vi "nejistota_A.vi"(11 "Array":dbl[](array[numeric])) -> (2 "nejistota_A":dbl, 3 "mean":dbl)   [LabVIEW 2022 SP3]
uses:
  <vilib>/Analysis/baseanly.llb/Mean (DBL).vi
  <vilib>/Analysis/NI_AALBase.lvlib
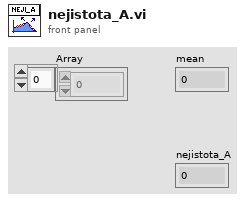
[diagram p1: front panel]
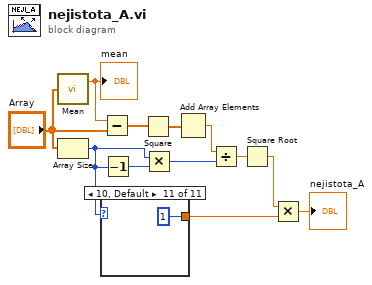
[diagram p0: block diagram]
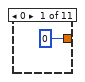
[diagram p2: hidden frame]
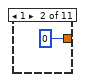
[diagram p3: hidden frame]
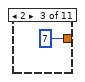
[diagram p4: hidden frame]
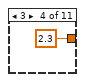
[diagram p5: hidden frame]
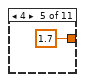
[diagram p6: hidden frame]
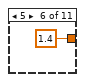
[diagram p7: hidden frame]
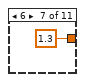
[diagram p8: hidden frame]
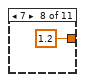
[diagram p9: hidden frame]
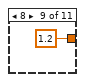
[diagram p10: hidden frame]
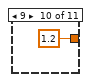
[diagram p11: hidden frame]
diagram:
  n1 = call-poly <vilib>:"Mean.vi"("X"="Array") -> ("mean"=w8:dbl)  [unwired: 1 out]
  "mean" <- w8
  n2 = Array Size(array="Array") -> (size(s)=w1:i32)
  n3 = case shown="10, Default" w1 {
    tunnel: [0 0 7 2.3 1.7 1.4 1.3 1.2 1.2 1.2 1] -> w7
    frame 0 {
    }
    frame 1 {
    }
    frame 2 {
    }
    frame 3 {
    }
    frame 4 {
    }
    frame 5 {
    }
    frame 6 {
    }
    frame 7 {
    }
    frame 8 {
    }
    frame 9 {
    }
    frame 10, Default {
    }
  }
  n4 = Subtract(x=w8, y="Array") -> (x-y=w9:dbl[])
  n5 = Decrement(x=w1) -> (x-1=w10:i32)
  n6 = Square(x=w9) -> (x^2=w4:dbl[])
  n7 = Multiply(x=w1, y=w10) -> (x*y=w11:i32)
  n8 = Add Array Elements(numeric array=w4) -> (sum=w3:dbl)
  n9 = Divide(x=w3, y=w11) -> (x/y=w12:dbl)
  n10 = Square Root(x=w12) -> (sqrt(x)=w6:dbl)
  n11 = Multiply(x=w6, y=w7) -> (x*y=→"nejistota_A":dbl)
